vi "checkNumRec.vi"(8 "error in (no error)":errorcluster, 11 "Logger in":refnum<class "Logger.lvclass">) -> (0 "error out":errorcluster, 2 "isToCreateNewFile":bool, 3 "Logger out":refnum<class "Logger.lvclass">)   [LabVIEW 2018, in "Logger.lvclass"]
doc: "Check the number of records to decide to generate the new log file or not."
uses:
  Logger.lvclass
  Logger.lvclass/Logger.ctl
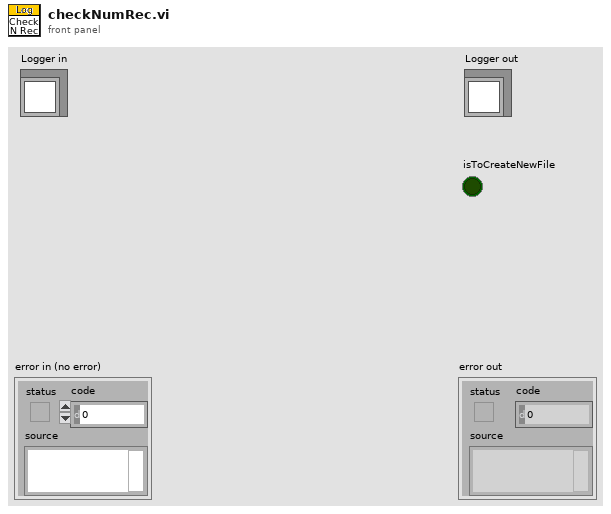
[diagram p1: front panel]
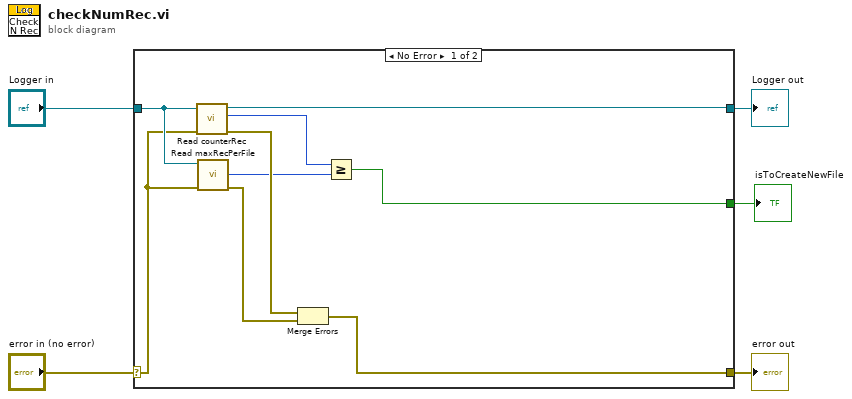
[diagram p0: block diagram]
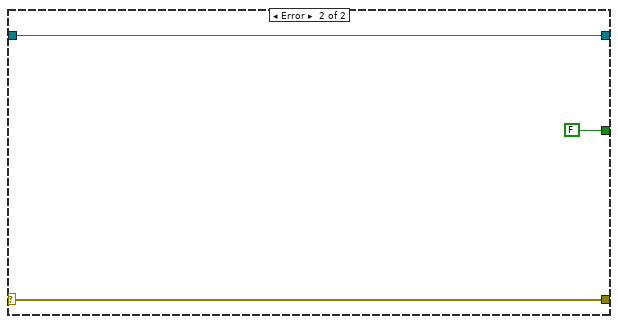
[diagram p2: hidden frame]
diagram:
  n1 = case shown="No Error" "error in (no error)" {
    selector: "error in (no error)" -> [w13 w17]
    tunnel: [w9 w17] -> w4
    tunnel: [w12 w16] -> w2
    tunnel: "Logger in" -> [w14 w16]
    tunnel: [w6 FALSE] -> w1
    frame No Error {
      n2 = call "Read counterRec.vi"("error in (no error)"=w13, "Logger in"=w14) -> ("error out"=w11:errorcluster, "counterRec"=w8:u32, "Logger out"=w12:refnum<class "Logger.lvclass">)  [unwired: 7 in]
      n3 = call "Read maxRecPerFile.vi"("error in (no error)"=w13, "Logger in"=w14) -> ("error out"=w10:errorcluster, "maxRecPerFile"=w7:u32)  [unwired: 7 in, 1 out]
      n4 = Merge Errors(w11, w10) -> (w9:errorcluster)
      n5 = Greater Or Equal?(x=w8, y=w7) -> (x >= y?=w6:bool)
    }
    frame Error {
    }
  }
  "error out" <- w4
  "Logger out" <- w2
  "isToCreateNewFile" <- w1
